vi "Attach Test Case.vi"(6 "Raw Results":T1[][](array[typedef]), 8 "error in (no error)":errorcluster, 9 "Result Indicies":cluster{"row":i32, "column":i32}[](array[cluster]), 10 "Testsuite Ref in":refnum<k20>, 11 "File Ref in":refnum<k20>) -> (0 "error out":errorcluster, 2 "Testsuite Ref out":refnum<k20>, 3 "File Ref out":refnum<k20>)   [LabVIEW 2014, in "VI Analyzer Parsing.lvlib"]
uses:
  VI Analyzer Parsing.lvlib
  <vilib>/addons/analyzer/_analyzerctrls.llb/VIAnCtl Results.ctl
  <vilib>/addons/analyzer/_analyzerctrls.llb/VIAnCtl ResultsData (index).ctl
  <vilib>/addons/analyzer/_analyzerctrls.llb/VIAnCtl ResultStatus.ctl
  <vilib>/ni/JUnit Results API/Controls/Test Case Attributes.ctl
  <vilib>/ni/JUnit Results API/Controls/Outcome Attributes.ctl
  <vilib>/xml/Close Reference(Node).vi
  <vilib>/ni/JUnit Results API/JUnit API.lvlib
  <vilib>/xml/NI_XML.lvlib
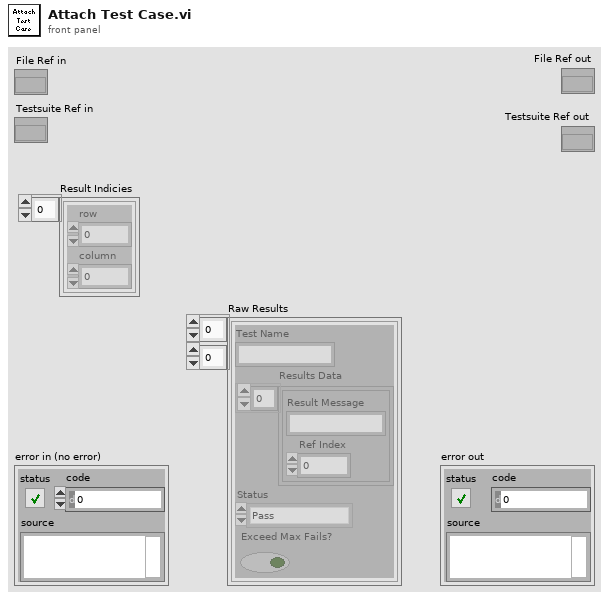
[diagram p1: front panel]
types:
  T1 = typedef "VIAnCtl Results.ctl" = cluster{"Test Name":string, "Results Data":T2[], "Status":T3, "Exceed Max Fails?":bool}
  T2 = typedef "VIAnCtl ResultsData (index).ctl" = cluster{"Result Message":string, "Ref Index":i32}
  T3 = typedef "VIAnCtl ResultStatus.ctl" = enum16{"Pass", "Fail", "Skipped", "VI not loadable", "Test not loadable", "Test not runnable", "Test error out"}
  T4 = typedef "JUnit API.lvlib/Test Case Attributes.ctl" = cluster{"name":string, "assertions":i32, "time":dbl, "timestamp":dbl, "classname":string, "status":string, "class":string, "file":string, "line":string, "log":string, "group":string, "url":string}
  T5 = typedef "JUnit API.lvlib/Outcome Attributes.ctl" = cluster{"message":string, "type":string}
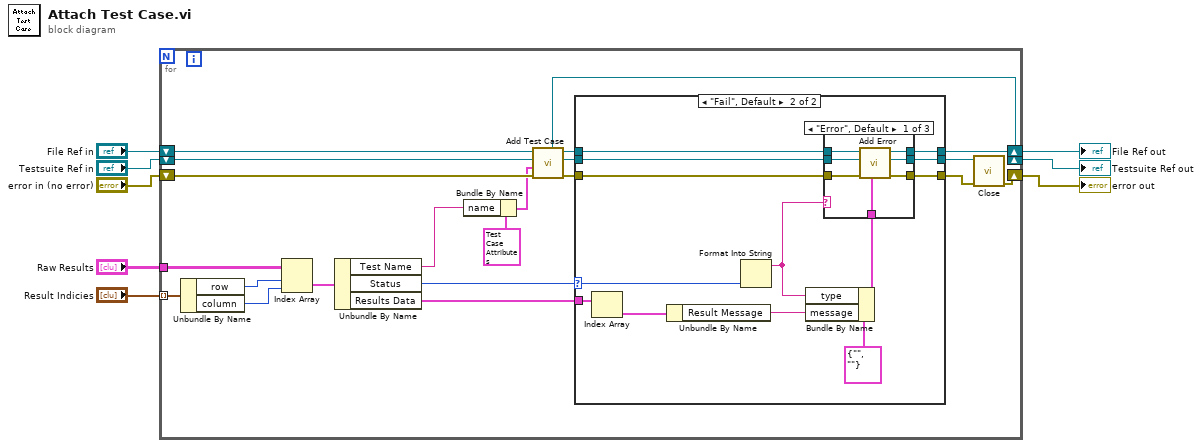
[diagram p0: block diagram]
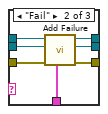
[diagram p3: hidden frame]
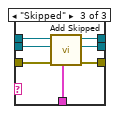
[diagram p4: hidden frame]
diagram:
  n1 = for {
    shift-right: [w19] -> w1
    shift-left: "error in (no error)" -> [w29]
    shift-right: [w22] -> w6
    shift-left: "Testsuite Ref in" -> [w27]
    shift-right: [w23] -> w5
    shift-left: "File Ref in" -> [w26]
    tunnel: "Result Indicies" -> [w16] mode=indexing
    tunnel: "Raw Results" -> [w15]
    n2 = Unbundle By Name(w16) -> ("row"=w14:i32, "column"=w9:i32)
    n3 = Index Array(array=w15, index (row)=w14, index (col)=w9) -> (element=w13:T1)
    n4 = Unbundle By Name(w13) -> ("Test Name"=w12:string, "Status"=w10:T3, "Results Data"=w11:T2[])
    n5 = Bundle By Name(cluster=T4 {"name"="", "assertions"=-1, "time"=-1.0, "timestamp"=-1.0, "classname"="", "status"="", "class"="", "file"="", "line"="", "log"="", "group"="", "url"=""} ("Test Case Atrributes"), "name"=w12) -> (w17:T4)
    n6 = call <vilib>:"Add Test Case.vi"("Error In (No Error)"=w29, "Test Case Atrributes"=w17, "Testsuite Ref In"=w27, "File Ref In"=w26) -> ("error out"=w28:errorcluster, "Testcase Ref"=w25:refnum<k20>, "File Ref Out"=w24:refnum<k20>, "Testsuite Ref Out"=w22:refnum<k20>)  [unwired: 4 in]
    n7 = case shown="\"Fail\", Default" w10 {
      selector: w10 -> [_ w35]
      tunnel: w28 -> [w30 w45]
      tunnel: w25 -> [w31 w44]
      tunnel: w24 -> [w32 w43]
      tunnel: [w32 w42] -> w23
      tunnel: [w31 w41] -> w21
      tunnel: [w30 w40] -> w20
      tunnel: w11 -> [_ w39]
      frame "Pass" {
      }
      frame "Fail", Default {
        n8 = Index Array(array=w39) -> (element=w38:T2)  [unwired: 1 in]
        n9 = Unbundle By Name(w38) -> ("Result Message"=w37:string)
        n10 = Format Into String(w35) -> (resulting string=w33:string)  [unwired: 3 in, 1 out]
        n11 = Bundle By Name(cluster=T5 {"message"="", "type"=""} ("Failure Attributes"), "type"=w33, "message"=w37) -> (w36:T5)
        n12 = case shown="\"Error\", Default" w33 {
          tunnel: w45 -> [w50 w59 w64]
          tunnel: w44 -> [w51 w58 w65]
          tunnel: w43 -> [w52 w57 w66]
          tunnel: [w49 w56 w61] -> w42
          tunnel: [w48 w55 w62] -> w41
          tunnel: [w47 w54 w63] -> w40
          tunnel: w36 -> [w46 w53 w60]
          frame "Error", Default {
            n13 = call <vilib>:"Add Error.vi"("Outcome Attributes"=w46, "Error In (No Error)"=w50, "Testcase Ref"=w51, "File Ref In"=w52) -> ("Error Out"=w47:errorcluster, "Testcase Ref Out"=w48:refnum<k20>, "File Ref Out"=w49:refnum<k20>)  [unwired: 5 in]
          }
          frame "Fail" {
            n14 = call <vilib>:"Add Failure.vi"("Outcome Attributes"=w53, "Error In (No Error)"=w59, "Testcase Ref"=w58, "File Ref In"=w57) -> ("Error Out"=w54:errorcluster, "Testcase Ref Out"=w55:refnum<k20>, "File Ref Out"=w56:refnum<k20>)  [unwired: 5 in]
          }
          frame "Skipped" {
            n15 = call <vilib>:"Add Skipped.vi"("Outcome Attributes"=w60, "Error In (No Error)"=w64, "Testcase Ref"=w65, "File Ref In"=w66) -> ("Error Out"=w63:errorcluster, "Testcase Ref Out"=w62:refnum<k20>, "File Ref Out"=w61:refnum<k20>)  [unwired: 5 in]
          }
        }
      }
    }
    n16 = call-poly <vilib>:"Close.vi"("error in (no error)"=w20, "node"=w21) -> ("error out"=w19:errorcluster)  [unwired: 7 in]
  }
  "Testsuite Ref out" <- w6
  "error out" <- w1
  "File Ref out" <- w5
